vi "Add Object.vi"   [LabVIEW 2020, in "NI_3D Picture Control.lvlib"]
doc: "Adds a 3D object to a scene."
uses:
  <vilib>/picture/3D Picture Control/NI_3D Picture Control.lvlib
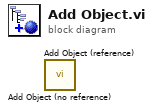
[diagram p0: block diagram]
diagram:
  n1 = call <vilib>:"Add Object (no reference).vi"() -> ()  [unwired: 10 in, 2 out]
  n2 = call <vilib>:"Add Object (reference).vi"() -> ()  [unwired: 9 in, 3 out]
